vi "Set JSON Config.vi"(8 "error in (no error)":errorcluster, 10 "<JSON>Config>":string, 11 "CFG Base in":refnum<class "CFG JSON.lvclass">) -> (0 "error out":errorcluster, 3 "CFG Base out":refnum<class "CFG JSON.lvclass">)   [LabVIEW 2023, in "HAL GOOP4.lvlib" / "CFG JSON.lvclass"]
uses:
  CFG JSON.lvclass
  CFG JSON.lvclass/CFG JSON.ctl
  <vilib>/JDP Science/JSONtext/JSONtext.lvlib
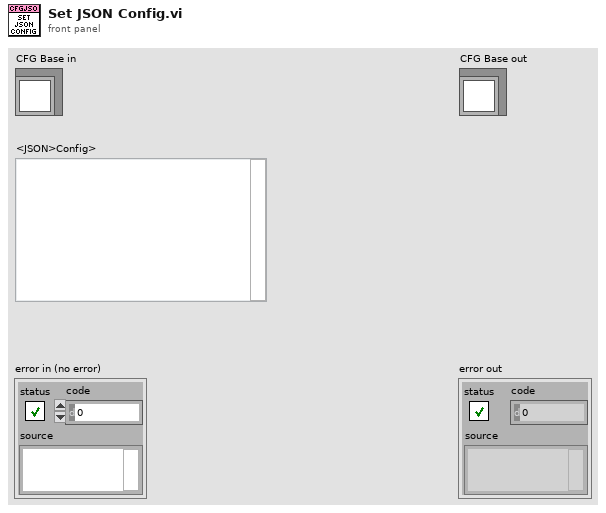
[diagram p1: front panel]
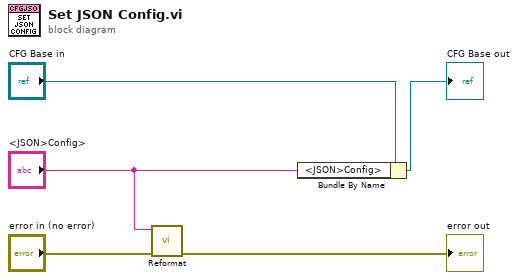
[diagram p0: block diagram]
diagram:
  n1 = call <vilib>:"Reformat.vi"("error in (no error)"="error in (no error)", "JSON"="<JSON>Config>") -> ("error out"=→"error out":errorcluster)  [unwired: 6 in, 3 out]
  n2 = Bundle By Name(cluster="CFG Base in", "<JSON>Config>"="<JSON>Config>") -> (→"CFG Base out":refnum<class "CFG JSON.lvclass">)
